vi "Test write VI RGB.vi"() -> ()   [LabVIEW 2023]
uses:
  gfitsio.lvlib
panel:
  out "error out":errorcluster
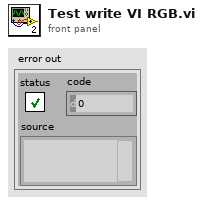
[diagram p1: front panel]
types:
  T1 = enum16{"diagram", "panel", ".vi file", "diagram, panel", "diagram, .vi file", "panel, .vi file", "diagram, panel, .vi file"}
  T2 = typedef "gfitsio.lvlib/gfitsio-refnum.ctl" = refnum<k1>
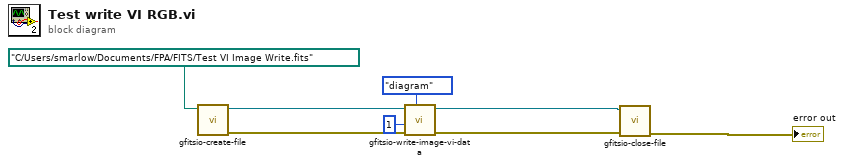
[diagram p0: block diagram]
diagram:
  n1 = call "gfitsio-create-file.vi"("path"=path "C:/Users/smarlow/Documents/FPA/FITS/Test VI Image Write.fits") -> ("error out"=w6:errorcluster, "gfits refnum"=w7:T2)  [unwired: 9 in]
  n2 = call "gfitsio-write-image-vi-data.vi"("requested data"=T1."diagram", "error in (no error)"=w6, "vi depth (1)"=1, "gfits refnum"=w7) -> ("error out"=w2:errorcluster, "dup gfits refnum"=w3:T2)  [unwired: 6 in]
  n3 = call "gfitsio-close-file.vi"("error in (no error)"=w2, "gfits refnum"=w3) -> ("error out"=→"error out":errorcluster)  [unwired: 8 in, 1 out]
